vi "HKey Classes Root Key Read Str.vi"(4 "error in (no error)":errorcluster, 5 "registry view":T1 items=["Default"=0, "KEY_WOW64_64KEY"=8, "KEY_WOW64_32KEY"=9], 6 "registry search value":string, 7 "registry search key":string) -> (0 "error out":errorcluster, 3 "result of registry search":string)   [LabVIEW 2017]
doc: "Read access to a DIAdem registry entry."
uses:
  <vilib>/registry/registry.llb/Registry View.ctl
  <vilib>/registry/registry.llb/Read Registry Value STR.vi
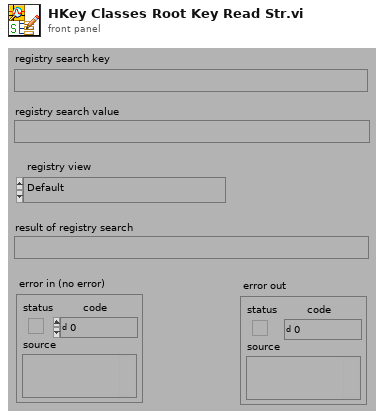
[diagram p1: front panel]
types:
  T1 = typedef "Registry View.ctl" = u16
  T2 = enum16{"KEY_QUERY_VALUE", "KEY_SET_VALUE", "KEY_CREATE_SUB_KEY", "KEY_ENUMERATE_SUB_KEYS", "KEY_NOTIFY", "KEY_CREATE_LINK", "KEY_READ", "KEY_WRITE", "KEY_ALL_ACCESS"}
  T3 = enum16{"HKEY_CLASSES_ROOT", "HKEY_CURRENT_USER", "HKEY_LOCAL_MACHINE", "HKEY_USERS", "HKEY_PERFORMANCE_DATA", "HKEY_CURRENT_CONFIG", "HKEY_DYN_DATA"}
  T4 = typedef "Registry refnum.ctl" = refnum<k1>
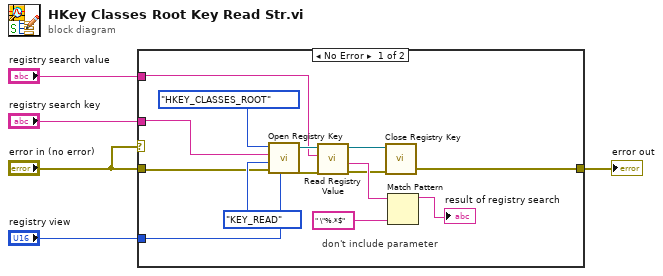
[diagram p0: block diagram]
diagram:
  n1 = case shown="No Error" "error in (no error)" {
    tunnel: "registry search key" -> [w10 _]
    tunnel: "registry search value" -> [w11 _]
    tunnel: "error in (no error)" -> [w9 w20]
    tunnel: [w8 w20] -> w2
    tunnel: "registry view" -> [w6 _]
    frame No Error {
      # "don't include parameter"
      n2 = call <vilib>:"Open Registry Key.vi"("registry view"=w6, "error in (no error)"=w9, "security access mask (KEY_READ | KEY_WRITE)"=T2."KEY_READ" ("security access mask (all)"), "subkey"=w10, "root key (HKEY_LOCAL_MACHINE)"=T3."HKEY_CLASSES_ROOT" ("root key")) -> ("error out"=w15:errorcluster, "refnum out"=w16:T4)  [unwired: 5 in]
      n3 = call-poly <vilib>:"Read Registry Value.vi"("error in (no error)"=w15, "value"=w11, "refnum"=w16) -> ("error out"=w12:errorcluster, "String/Binary data"=w14:string, "refnum out"=w13:T4)  [unwired: 5 in, 1 out]
      n4 = call <vilib>:"Close Registry Key.vi"("error in (no error)"=w12, "refnum"=w13) -> ("error out"=w8:errorcluster)  [unwired: 5 in]
      n5 = Match Pattern(string=w14, regular expression=" \"%.*$") -> (before substring=→"result of registry search":string)  [unwired: 1 in, 3 out]
    }
    frame Error {
    }
  }
  "error out" <- w2
